vi "Terminal Test.vi"() -> ()   [LabVIEW 2020, in "Serial Test.lvlib"]
uses:
  Serial Test.lvlib
  Stream-Serial/Serial Client/Serial Client.lvclass
  <vilib>/IlluminatedG/lv-stream/Endpoint/Endpoint.lvclass
  <vilib>/IlluminatedG/lv-stream/Connection/Connection.lvclass
  <vilib>/IlluminatedG/lv-stream/Connection/State.ctl
  <vilib>/IlluminatedG/lv-stream/stream/Stream.lvclass
  C:/Program Files (x86)/National Instruments/LabVIEW 2020/vi.lib/IlluminatedG/lv-stream/Connection/Connection.lvclass
  C:/Program Files (x86)/National Instruments/LabVIEW 2020/vi.lib/IlluminatedG/lv-stream/Endpoint/Endpoint.lvclass
  Stream-Serial/Serial Client/Stop Bits.ctl
  Stream-Serial/Serial Client/Flow Control.ctl
  Stream-Serial/Serial Client/Parity.ctl
  Stream-Serial/Serial Client/Port Config.ctl
panel:
  in  "Close":bool
  in  "Open":bool
  out "Log":string
  out "Connected":bool
  in  "Port Config (115200 8N1)":T1={"Baud (115200)"=115200, "Data Bits (8)"=8, "Stop Bits (1)"=10, "Flow Control"=0, "Use LineTerm?"=FALSE, "LineTerm (\\n)"="\n", "Timeout ms (10000)"=10000, "Parity (None)"=enum."None"} {"Flow Control" items=["None", "XON/XOFF", "RTS/CTS", "XON/XOFF & RTS/CTS", "DTR/DSR", "XON/XOFF & DTR/DSR"]; "Stop Bits (1)" items=["1.0"=10, "1.5"=15, "2.0"=20]}
  in  "Serial Port":refnum<visa-resource-name>
  # "Select the Port and choose the config before running the VI"
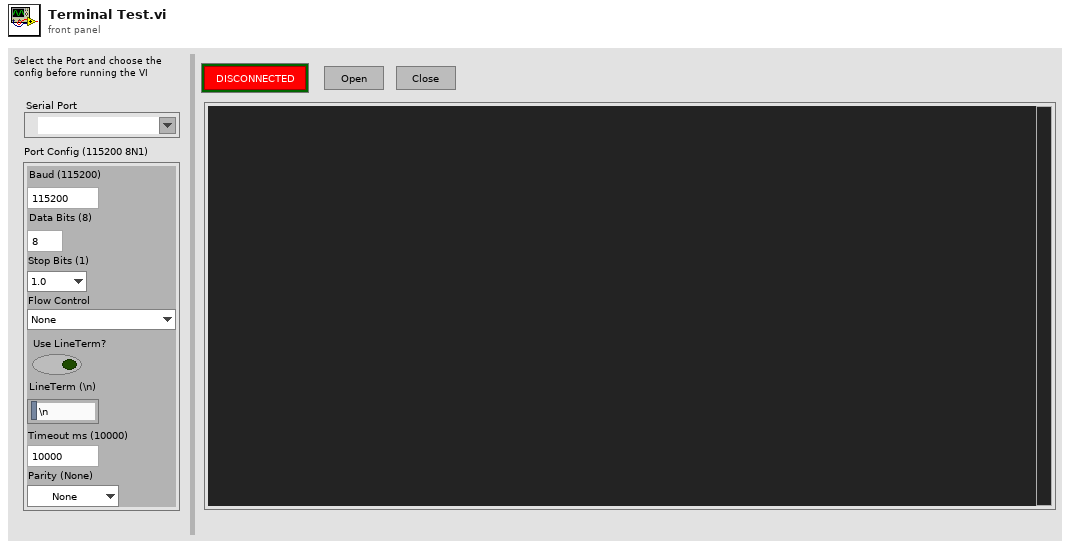
[diagram p1: front panel]
types:
  T1 = typedef "Stream-Serial.lvlib/Serial Client.lvclass/Port Config.ctl" = cluster{"Baud (115200)":u32, "Data Bits (8)":u8, "Stop Bits (1)":T2, "Flow Control":T3, "Use LineTerm?":bool, "LineTerm (\\n)":string, "Timeout ms (10000)":i32, "Parity (None)":T4}
  T2 = typedef "Stream-Serial.lvlib/Serial Client.lvclass/Stop Bits.ctl" = u16
  T3 = typedef "Stream-Serial.lvlib/Serial Client.lvclass/Flow Control.ctl" = u16
  T4 = typedef "Stream-Serial.lvlib/Serial Client.lvclass/Parity.ctl" = enum16{"None", "Odd", "Even", "Mark", "Space"}
  T5 = typedef "Stream.lvlib/Connection.lvclass/State.ctl" = enum16{"Closed", "Idle", "Connecting", "Connected", "Shutdown"}
  T6 = typedef "eventvkey.ctl" = enum16{"ASCII", "Enter", "Return", "Shift", "Ctrl", "Alt", "Cmd", "Opt", "Caps", "NumLock", "Clear", "Break", "Up", "Down", "Left", "Right", "Insert", "Delete", "Home", "End", "PageUp", "PageDown", "Escape", "Help", "Pause", "ScrollLock", "F1", "F2", "F3", "F4", "F5", "F6", "F7", "F8", "F9", "F10", "F11", "F12", "F13", "F14", "F15", "F16", "F17", "F18", "F19", "F20", "F21", "F22", "F23", "F24", "Play", "VolumeUp", "VolumeDown", "Mute", "Two Byte Char"}
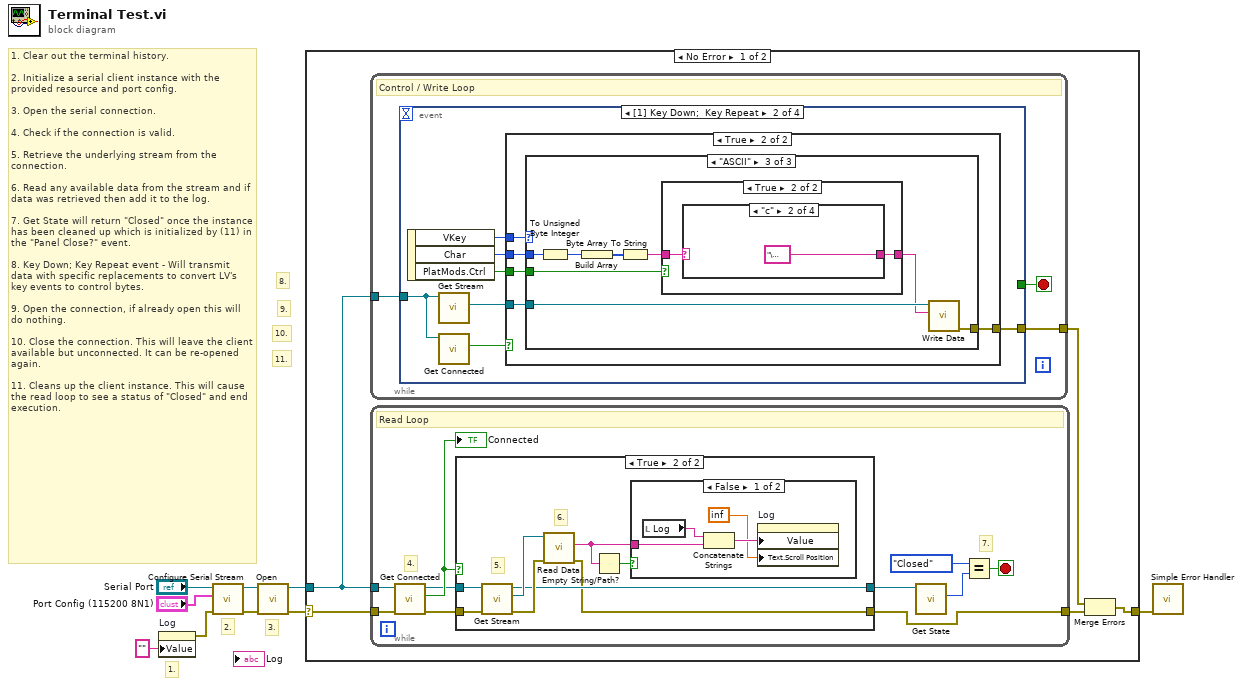
[diagram p0: block diagram]
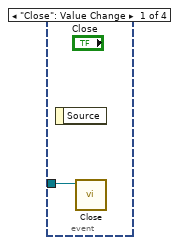
[diagram p2: hidden frame]
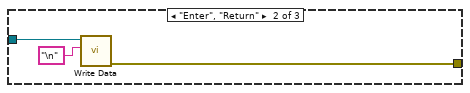
[diagram p5: hidden frame]
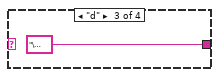
[diagram p8: hidden frame]
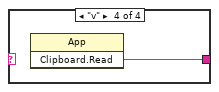
[diagram p9: hidden frame]
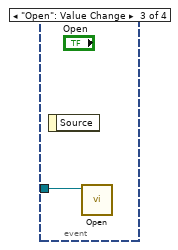
[diagram p10: hidden frame]
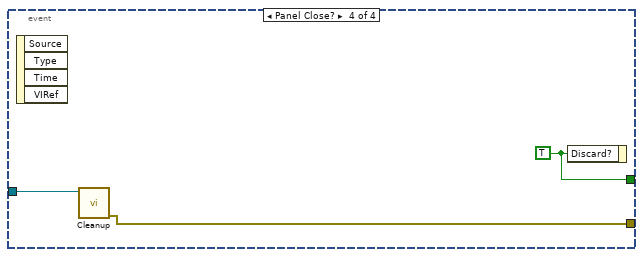
[diagram p11: hidden frame]
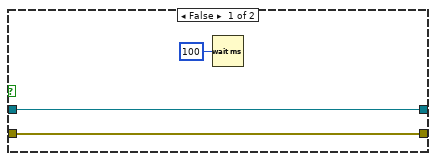
[diagram p12: hidden frame]
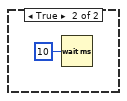
[diagram p13: hidden frame]
diagram:
  # "11."
  # "10."
  # "9."
  # "8."
  # "3."
  # "2."
  # "1."
  # "1. Clear out the terminal history.\n\n2. Initialize a serial client instance with the provided resource and port config.\n\n3. Open the serial connection.\n\n4. Check if the connection is valid.\n\n5. Retrieve the underlying stream from the connection.\n\n6. Read any available data from the stream and if data was retrieved then add it to the log.\n\n7. Get State will return \"Closed\" once the instance has been cleaned up which is initialized by (11) in the \"Panel Close?\" event.\n\n8. Key Down; Key Repeat event - Will transmit data with specific replacements to convert LV's key events to control bytes.\n\n9. Open the connection, if already open this will do nothing.\n\n10. Close the connection. This will leave the client available but unconnected. It can be re-opened again.\n\n11. Cleans up the client instance. This will cause the read loop to see a status of \"Closed\" and end execution."
  n1 = property on="Log" class="Str"("Value"="" ("Log")) -> (error out=w7:errorcluster)  [unwired: 2 in, 1 out]
  n2 = call "Configure Serial Stream.vi"("error in (no error)"=w7, "Port Config (115200 8N1)"="Port Config (115200 8N1)", "Serial Port"="Serial Port") -> ("error out"=w3:errorcluster, "Serial Client out"=w4:refnum<class "Serial Client.lvclass">)  [unwired: 7 in]
  n3 = call <vilib>:"Open.vi"("error in (no error)"=w3, "Endpoint in"=w4) -> ("error out"=w2:errorcluster, "Endpoint out"=w1:refnum<class "Serial Client.lvclass">)  [unwired: 8 in]
  n4 = case shown="No Error" w2 {
    selector: w2 -> [w14 w79]
    tunnel: w1 -> [w13 _]
    tunnel: [w12 w79] -> w5
    frame No Error {
      n5 = while {
        tunnel: w13 -> [w16]
        tunnel: [w15] -> w10
        stop <- w17 stop-if-true
        # "Control / Write Loop"
        n6 = event shown="[1] Key Down;  Key Repeat" {
          selector: _ -> [_ _ _ _]
          dyn-events: _ -> [_ _ _ _]
          timeout: _ -> [_ _ _ _]
          tunnel: w16 -> [w18 w20 w49 w51]
          tunnel: [_ _ _ w52] -> w17
          tunnel: [_ w22 _ w50] -> w15
          event "Close": Value Change {
            n7 = event-data() -> ()  [unwired: 1 in, 1 out]
            n8 = call <vilib>:"Close.vi"("Endpoint in"=w18) -> ()  [unwired: 9 in, 2 out]
          }
          event Key Down; Key Repeat {
            n9 = event-data() -> ("VKey"=w19:T6, "Char"=w24:i16, "PlatMods.Ctrl"=w25:bool)  [unwired: 1 in]
            n10 = call-dynamic "Get Stream.vi"("VISA Client in"=w20) -> ("Stream"=w23:refnum<class "Stream.lvclass">)  [unwired: 8 in, 2 out]
            n11 = call <vilib>:"Get Connected.vi"("Connection in"=w20) -> ("Connected"=w21:bool)  [unwired: 8 in, 2 out]
            n12 = case shown="True" w21 {
              tunnel: w25 -> [_ w27]
              tunnel: w24 -> [_ w30]
              tunnel: w23 -> [_ w29]
              tunnel: [_ w28] -> w22
              tunnel: w19 -> [_ w26]
              frame False {
              }
              frame True {
                n13 = case shown="\"ASCII\"" w26 {
                  tunnel: w30 -> [_ _ w41]
                  tunnel: w29 -> [_ w33 w36]
                  tunnel: [_ w32 w34] -> w28
                  tunnel: w27 -> [_ _ w37]
                  frame Default {
                  }
                  frame "Enter", "Return" {
                    n14 = call <vilib>:"Write Data.vi"("Data"="\n", "Stream in"=w33) -> ("error out"=w32:errorcluster)  [unwired: 8 in, 1 out]
                  }
                  frame "ASCII" {
                    n15 = To Unsigned Byte Integer(number=w41) -> (unsigned 8bit integer=w40:u8)
                    n16 = Build Array(w40) -> (w39:u8[])
                    n17 = Byte Array To String(unsigned byte array=w39) -> (string=w38:string)
                    n18 = case shown="True" w37 {
                      tunnel: w38 -> [w42 w44]
                      tunnel: [w42 w43] -> w35
                      frame False {
                      }
                      frame True {
                        n19 = case shown="\"c\"" w44 {
                          selector: w44 -> [w45 _ _ _]
                          tunnel: [w45 "\u0003" ("Data") "\u0004" ("Data") w48] -> w43
                          frame Default {
                          }
                          frame "c" {
                          }
                          frame "d" {
                          }
                          frame "v" {
                            n20 = invoke class="App" method="Clipboard.Read"() -> ("Read Clipbrd"=w48:string)  [unwired: 3 in, 2 out]
                          }
                        }
                      }
                    }
                    n21 = call <vilib>:"Write Data.vi"("Data"=w35, "Stream in"=w36) -> ("error out"=w34:errorcluster)  [unwired: 8 in, 1 out]
                  }
                }
              }
            }
          }
          event "Open": Value Change {
            n22 = event-data() -> ()  [unwired: 1 in, 1 out]
            n23 = call <vilib>:"Open.vi"("Endpoint in"=w49) -> ()  [unwired: 9 in, 2 out]
          }
          event Panel Close? {
            w52 = TRUE ("Discard?")
            n24 = event-data() -> ()  [unwired: 1 in, 4 out]
            n25 = call-dynamic "Cleanup.vi"("VISA Client in"=w51) -> ("error out"=w50:errorcluster)  [unwired: 10 in]
            n26 = event-data("Discard?"=w52) -> ()  [unwired: 1 in, 1 out]
          }
        }
      }
      n27 = while {
        tunnel: w13 -> [w62]
        tunnel: w14 -> [w61]
        tunnel: [w53] -> w11
        stop <- w57 stop-if-true
        # "7."
        # "4."
        # "Read Loop"
        n28 = call <vilib>:"Get Connected.vi"("error in (no error)"=w61, "Connection in"=w62) -> ("error out"=w60:errorcluster, "Connected"=w59:bool, "Connection out"=w58:refnum<class "Serial Client.lvclass">)  [unwired: 7 in]
        "Connected" <- w59
        n29 = case shown="True" w59 {
          tunnel: w58 -> [w65 w73]
          tunnel: w60 -> [w64 w72]
          tunnel: [w65 w67] -> w56
          tunnel: [w64 w66] -> w53
          frame False {
            n30 = Wait (ms)(milliseconds to wait=u32 100) -> ()  [unwired: 1 out]
          }
          frame True {
            # "6."
            # "5."
            n31 = call-dynamic "Get Stream.vi"("error in (no error)"=w72, "VISA Client in"=w73) -> ("error out"=w70:errorcluster, "Stream"=w71:refnum<class "Stream.lvclass">, "VISA Client out"=w67:refnum<class "Serial Client.lvclass">)  [unwired: 7 in]
            n32 = call <vilib>:"Read Data.vi"("error in (no error)"=w70, "Stream in"=w71) -> ("error out"=w66:errorcluster, "Data"=w69:string)  [unwired: 7 in, 1 out]
            n33 = Empty String/Path?(string/path=w69) -> (empty?=w68:bool)
            n34 = case shown="False" w68 {
              tunnel: w69 -> [w74 _]
              frame False {
                n35 = local read "Log"() -> (w77:string)
                n36 = Concatenate Strings(w77, w74) -> (w76:string)
                n37 = property on="Log" class="Str"("Value"=w76, "Text.Scroll Position"=inf) -> ()  [unwired: 2 in, 2 out]
              }
              frame True {
                n38 = Wait (ms)(milliseconds to wait=u32 10) -> ()  [unwired: 1 out]
              }
            }
          }
        }
        n39 = call <vilib>:"Get State.vi"("Connection in"=w56) -> ("State"=w55:T5)  [unwired: 8 in, 2 out]
        n40 = Equal?(x=State."Closed", y=w55) -> (x = y?=w57:bool)
      }
      n41 = Merge Errors(w10, w11) -> (w12:errorcluster)
    }
    frame Error {
    }
  }
  n42 = call <vilib>:"Simple Error Handler.vi"("error in (no error)"=w5) -> ()  [unwired: 4 in, 5 out]
